vi "ex_Validate String.vi"(0 "VI Refnum":refnum<vi>, 5 "Old Val":string, 7 "New Val":string, 9 "Str Refnum":refnum<vi>, 12 "Allow Empty String?":bool, 13 "Exceptions":string[](array[string]), 14 "Additional Prohibited Strings":string[](array[string])) -> (4 "Val Out":string, 6 "Name Conflict":bool)   [LabVIEW 2020]
panel:
  out "Invalid Text":string
  in  "Empty String":string="<< Empty String >>"
  in  "Close":bool
  out "Message":string="The text you entered is not allowed because it is reserved for this Express VI. You must change the text so that it does not include a value displayed in the following list of reserved text."
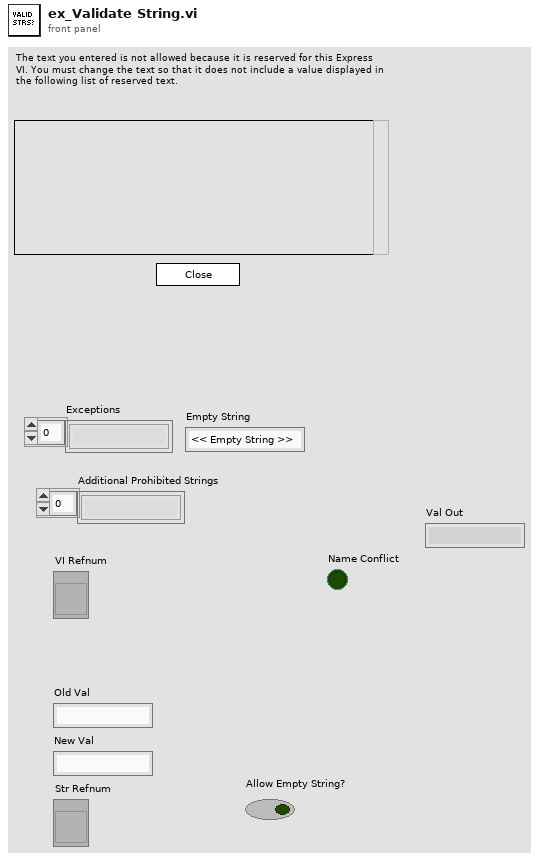
[diagram p1: front panel]
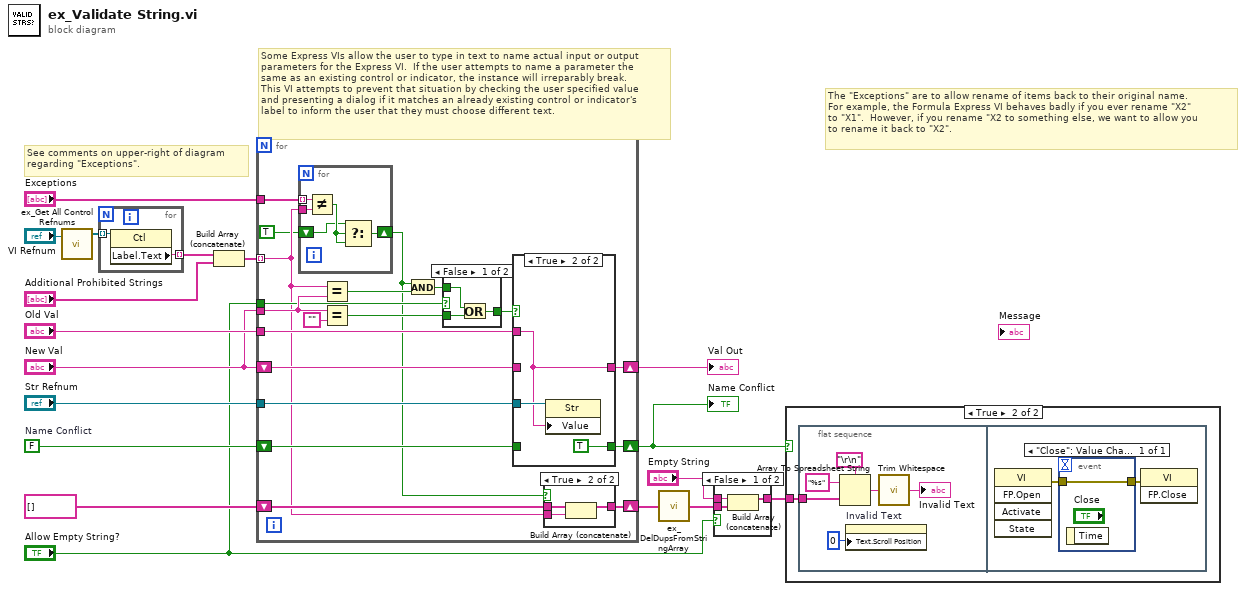
[diagram p0: block diagram]
diagram:
  w15 = FALSE  # Name Conflict
  # "See comments on upper-right of diagram\nregarding \"Exceptions\"."
  # "The \"Exceptions\" are to allow rename of items back to their original name.\nFor example, the Formula Express VI behaves badly if you ever rename \"X2\"\nto \"X1\".  However, if you rename \"X2 to something else, we want to allow you\nto rename it back to \"X2\"."
  # "Some Express VIs allow the user to type in text to name actual input or output\nparameters for the Express VI.  If the user attempts to name a parameter the\nsame as an existing control or indicator, the instance will irreparably break.\nThis VI attempts to prevent that situation by checking the user specified value\nand presenting a dialog if it matches an already existing control or indicator's\nlabel to inform the user that they must choose different text."
  n1 = call <vilib>:"ex_Get All Control Refnums.vi"("viref Express VI"="VI Refnum") -> ("All Controls[]"=w5:refnum<vi>[])  [unwired: 2 in, 1 out]
  n2 = for {
    tunnel: w5 -> [w20] mode=indexing
    tunnel: [w19] -> w4 mode=indexing
    n3 = property class="Ctl"(reference=w20) -> ("Label.Text"=w19:string)  [unwired: 1 in, 2 out]
  }
  n4 = Build Array (concatenate)(w4, "Additional Prohibited Strings") -> (w3:string[])
  n5 = for {
    shift-right: [w38] -> w7
    shift-left: string[] [] -> [w39]
    tunnel: "Str Refnum" -> [w37]
    shift-right: [w34] -> w14
    shift-left: "New Val" -> [w36]
    tunnel: "Old Val" -> [w35]
    shift-right: [w32] -> w13
    shift-left: w15 -> [w33]
    tunnel: "New Val" -> [w31]
    tunnel: "Allow Empty String?" -> [w29]
    tunnel: "Exceptions" -> [w26]
    tunnel: w3 -> [w23] mode=indexing
    n6 = for {
      tunnel: w26 -> [w44] mode=indexing
      tunnel: w23 -> [w43]
      shift-right: [w42] -> w21
      shift-left: TRUE -> [w40]
      n7 = Not Equal?(x=w44, y=w43) -> (x != y?=w41:bool)
      n8 = Select(t=w40, s=w41, f=w41) -> (s? t:f=w42:bool)
    }
    n9 = Equal?(x=w23, y=w31) -> (x = y?=w24:bool)
    n10 = Equal?(x=w31, y="") -> (x = y?=w27:bool)
    n11 = And(x=w21, y=w24) -> (x .and. y?=w25:bool)
    n12 = case shown="False" w29 {
      tunnel: [w51 w52] -> w28
      tunnel: w25 -> [w49 w52]
      tunnel: w27 -> [w50 _]
      frame False {
        n13 = Or(x=w49, y=w50) -> (x .or. y?=w51:bool)
      }
      frame True {
      }
    }
    n14 = case shown="True" w28 {
      tunnel: w37 -> [_ w57]
      tunnel: w36 -> [w54 _]
      tunnel: [w54 w56] -> w34
      tunnel: w35 -> [_ w56]
      tunnel: w33 -> [w53 _]
      tunnel: [w53 TRUE ("Name Conflict")] -> w32
      frame False {
      }
      frame True {
        n15 = property class="Str"(reference=w57, "Value"=w56) -> ()  [unwired: 1 in, 2 out]
      }
    }
    n16 = case shown="True" w21 {
      tunnel: w39 -> [w45 w48]
      tunnel: [w45 w47] -> w38
      tunnel: w23 -> [_ w46]
      frame False {
      }
      frame True {
        n17 = Build Array (concatenate)(w48, w46) -> (w47:string[])
      }
    }
  }
  "Val Out" <- w14
  "Name Conflict" <- w13
  n18 = call <vilib>:"ex_DelDupsFromStringArray.vi"("string array"=w7) -> ("String array without duplicates"=w6:string[])  [unwired: 13 in, 1 out]
  n19 = case shown="False" "Allow Empty String?" {
    tunnel: w6 -> [w60 w61]
    tunnel: "Empty String" -> [w59 _]
    tunnel: [w58 w61] -> w10
    frame False {
      n20 = Build Array (concatenate)(w59, w60) -> (w58:string[])
    }
    frame True {
    }
  }
  n21 = case shown="True" w13 {
    tunnel: w10 -> [_ w62]
    frame False {
    }
    frame True {
      n22 = flat-sequence {
        tunnel: w62 -> [w68]
        frame #0 {
          n23 = Array To Spreadsheet String(delimiter (Tab)="\r\n", array=w68, 3:"%s" ("format string")) -> (spreadsheet string=w64:string)
          n24 = property on="Invalid Text" class="Str"("Text.Scroll Position"=u32 0) -> ()  [unwired: 2 in, 2 out]
          n25 = call <vilib>:"Trim Whitespace.vi"("string"=w64) -> ("trimmed string"=→"Invalid Text":string)  [unwired: 1 in]
        }
        frame #1 {
          n26 = invoke class="VI" method="FP.Open"() -> (error out=w70:errorcluster)  [unwired: 5 in, 4 out]
          n27 = event shown="[0] \"Close\": Value Change" {
            selector: _ -> [_]
            dyn-events: _ -> [_]
            timeout: _ -> [_]
            tunnel: w70 -> [w71]
            tunnel: [w71] -> w69
            event "Close": Value Change {
              n28 = event-data() -> ()  [unwired: 1 in, 1 out]
            }
          }
          n29 = invoke class="VI" method="FP.Close"(error in=w69) -> ()  [unwired: 2 in, 3 out]
        }
      }
    }
  }
